vi "Test Process Broadcast Lifecycle Changes.vi"(8 "error in (no error)":errorcluster, 11 "Process Test In":refnum<class "Process Dev Test.lvclass">) -> (0 "error out":errorcluster, 3 "Process Test Out":refnum<class "Process Dev Test.lvclass">)   [LabVIEW 2020, in "Process Dev Test.lvclass"]
uses:
  Process Dev Test.lvclass
  C:/Program Files (x86)/National Instruments/LabVIEW 2020/vi.lib/Astemes/LUnit/Test Case.lvclass
  source/Framework/Process/Process.lvclass/Process.ctl
  <vilib>/Astemes/LUnit/Test Case.lvclass/Test Case.ctl
  <vilib>/Astemes/LUnit/LUnit Assertion Result.lvclass/LUnit Assertion Result.ctl
  <vilib>/Astemes/LUnit/LUnit Test Case Result.lvclass/LUnit Test Case Result.ctl
  <vilib>/Astemes/LUnit/LUnit Method Result.lvclass/LUnit Method Result.ctl
  source/Framework/Process/Public/Lifecycle/Get Lifecycle State.vi
  source/Framework/Broadcast Event Helpers/Execution timer.vi
  <vilib>/Astemes/LUnit/Palette/Fail.vi
  <vilib>/Astemes/LUnit/Palette/Pass.vi
  <vilib>/Astemes/LUnit/Set Assertion Type.vi
  source/Framework/Process/Private/SubVIs/Wait for finish.vi
  source/Framework/Process/Protected/Messaging/Enqueue Message.vi
  source/Framework/Process/Private/SubVIs/Set Lifecycle State.vi
  <vilib>/Utility/error.llb/Clear Errors.vi
  <vilib>/Astemes/LUnit/Add test result.vi
  <vilib>/Astemes/LUnit/LUnit Write Passed.vi
  <vilib>/Astemes/LUnit/LUnit Write Message.vi
  <vilib>/Astemes/LUnit/LUnit Write Description.vi
  <vilib>/Astemes/LUnit/LUnit Write Assertion Type.vi
  source/Framework/Process/Private/SubVIs/Handle Debug Data.vi
  <vilib>/Astemes/LUnit/LUnit Record Assertion Result.vi
  source/Framework/Logging/Log Debug.vi
  <vilib>/AdvancedString/1D String Array to Delimited String.vi
  <vilib>/Utility/High Resolution Relative Seconds.vi
  <vilib>/Astemes/LUnit/LUnit Aggregate Assertion Results.vi
  <vilib>/Astemes/LUnit/Assertion Result/LUnit Read Status.vi
  <vilib>/Astemes/LUnit/LUnit Read Message.vi
  <vilib>/Astemes/LUnit/LUnit Read Description.vi
  <vilib>/Astemes/LUnit/Method Result/LUnit Merge Status.vi
  <vilib>/Astemes/LUnit/LUnit Concatenate result strings.vi
  <vilib>/Utility/error.llb/Error Cluster From Error Code.vi
  source/Framework/Broadcast Event Helpers/Dequeue Broadcast Message.vi
  source/Framework/Process/Public/Read Name.vi
  <vilib>/Astemes/LUnit/LUnit Assertion Result.lvclass
  source/Framework/Process/Process.lvclass
  <vilib>/Astemes/LUnit/Test Case.lvclass
  source/Framework/Broadcast Event Helpers/Broadcast Event Helpers.lvlib
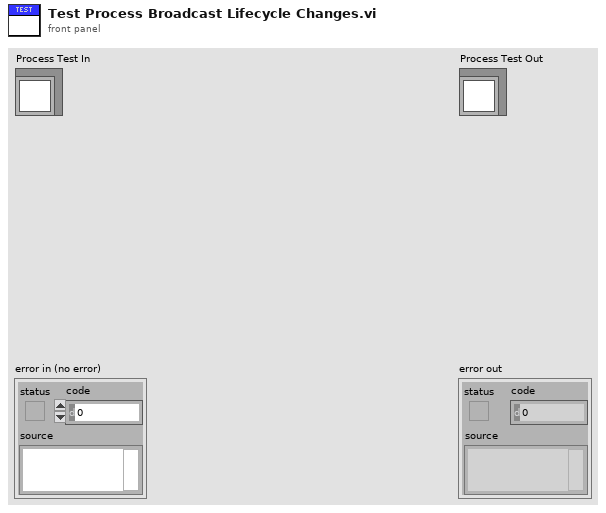
[diagram p1: front panel]
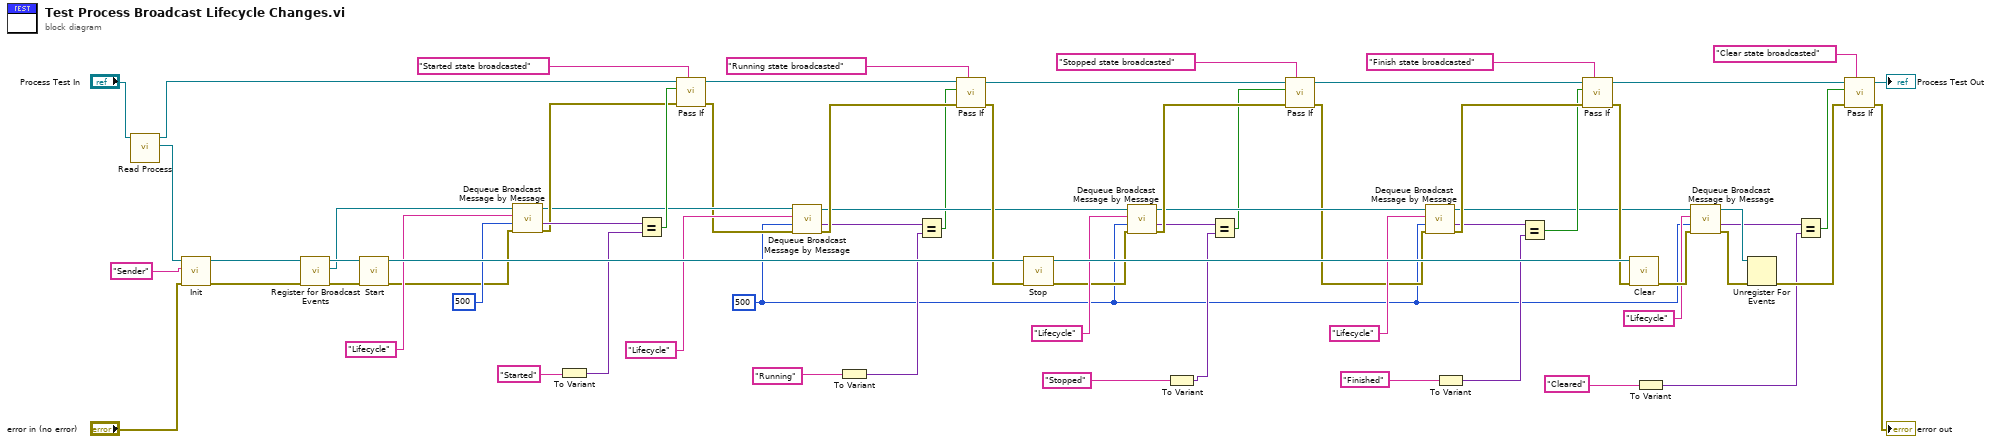
[diagram p0: block diagram]
diagram:
  w1 = 500
  n1 = call "Read Process.vi"("Process Test in"="Process Test In") -> ("Process.lvclass"=w62:refnum<class "Process.lvclass">, "Process Test out"=w21:refnum<class "Process Dev Test.lvclass">)  [unwired: 8 in, 1 out]
  n2 = call-dynamic "Init.vi"("error in (no error)"="error in (no error)", "Name"="Sender" ("Message"), "Process In"=w62) -> ("error out"=w67:errorcluster, "Process Out"=w68:refnum<class "Process.lvclass">)  [unwired: 7 in]
  n3 = call "Register for Broadcast Events.vi"("error in (no error)"=w67, "Process In"=w68) -> ("error out"=w60:errorcluster, "Event Registration Refnum Out"=w25:refnum<event-registration>, "Process Out"=w61:refnum<class "Process.lvclass">)  [unwired: 7 in]
  n4 = call "Start.vi"("error in (no error)"=w60, "Process In"=w61) -> ("error out"=w23:errorcluster, "Process Out"=w59:refnum<class "Process.lvclass">)  [unwired: 7 in, 1 out]
  n5 = call "Dequeue Broadcast Message by Message.vi"("error in (no error)"=w23, "Timeout (-1)"=500, "Message"="Lifecycle", "Event Registration Refnum"=w25) -> ("error out"=w27:errorcluster, "Message Data"=w28:variant, "Event Registration Refnum Out"=w24:refnum<event-registration>)  [unwired: 3 in, 2 out]
  n6 = To Variant(anything="Started") -> (Variant=w32:variant)
  n7 = Equal?(x=w28, y=w32) -> (x = y?=w31:bool)
  n8 = call <vilib>:"Pass If.vi"("Description"="Started state broadcasted", "error in (no error)"=w27, "Pass?"=w31, "LUnit Test Case In"=w21) -> ("error out"=w22:errorcluster, "LUnit Test Case Out"=w20:refnum<class "Process Dev Test.lvclass">)  [unwired: 6 in]
  n9 = call "Dequeue Broadcast Message by Message.vi"("error in (no error)"=w22, "Timeout (-1)"=w1, "Message"="Lifecycle", "Event Registration Refnum"=w24) -> ("error out"=w57:errorcluster, "Message Data"=w55:variant, "Event Registration Refnum Out"=w45:refnum<event-registration>)  [unwired: 3 in, 2 out]
  n10 = To Variant(anything="Running" ("Message")) -> (Variant=w38:variant)
  n11 = Equal?(x=w55, y=w38) -> (x = y?=w39:bool)
  n12 = call <vilib>:"Pass If.vi"("Description"="Running state broadcasted", "error in (no error)"=w57, "Pass?"=w39, "LUnit Test Case In"=w20) -> ("error out"=w56:errorcluster, "LUnit Test Case Out"=w41:refnum<class "Process Dev Test.lvclass">)  [unwired: 6 in]
  n13 = call "Stop.vi"("error in (no error)"=w56, "Process In"=w59) -> ("error out"=w43:errorcluster, "Process Out"=w66:refnum<class "Process.lvclass">)  [unwired: 7 in, 1 out]
  n14 = call "Dequeue Broadcast Message by Message.vi"("error in (no error)"=w43, "Timeout (-1)"=w1, "Message"="Lifecycle", "Event Registration Refnum"=w45) -> ("error out"=w49:errorcluster, "Message Data"=w47:variant, "Event Registration Refnum Out"=w44:refnum<event-registration>)  [unwired: 3 in, 2 out]
  n15 = To Variant(anything="Stopped" ("Message")) -> (Variant=w36:variant)
  n16 = Equal?(x=w47, y=w36) -> (x = y?=w37:bool)
  n17 = call <vilib>:"Pass If.vi"("Description"="Stopped state broadcasted", "error in (no error)"=w49, "Pass?"=w37, "LUnit Test Case In"=w41) -> ("error out"=w42:errorcluster, "LUnit Test Case Out"=w40:refnum<class "Process Dev Test.lvclass">)  [unwired: 6 in]
  n18 = call "Dequeue Broadcast Message by Message.vi"("error in (no error)"=w42, "Timeout (-1)"=w1, "Message"="Lifecycle", "Event Registration Refnum"=w44) -> ("error out"=w51:errorcluster, "Message Data"=w35:variant, "Event Registration Refnum Out"=w15:refnum<event-registration>)  [unwired: 3 in, 2 out]
  n19 = To Variant(anything="Finished" ("Message")) -> (Variant=w34:variant)
  n20 = Equal?(x=w35, y=w34) -> (x = y?=w33:bool)
  n21 = call <vilib>:"Pass If.vi"("Description"="Finish state broadcasted", "error in (no error)"=w51, "Pass?"=w33, "LUnit Test Case In"=w40) -> ("error out"=w50:errorcluster, "LUnit Test Case Out"=w11:refnum<class "Process Dev Test.lvclass">)  [unwired: 6 in]
  n22 = call-dynamic "Clear.vi"("error in (no error)"=w50, "Process In"=w66) -> ("error out"=w14:errorcluster)  [unwired: 9 in]
  n23 = To Variant(anything="Cleared" ("Message")) -> (Variant=w4:variant)
  n24 = call "Dequeue Broadcast Message by Message.vi"("error in (no error)"=w14, "Timeout (-1)"=w1, "Message"="Lifecycle", "Event Registration Refnum"=w15) -> ("error out"=w13:errorcluster, "Message Data"=w5:variant, "Event Registration Refnum Out"=w12:refnum<event-registration>)  [unwired: 3 in, 2 out]
  n25 = Unregister For Events(event registration refnum=w12, error in=w13) -> (error out=w9:errorcluster)
  n26 = Equal?(x=w5, y=w4) -> (x = y?=w3:bool)
  n27 = call <vilib>:"Pass If.vi"("Description"="Clear state broadcasted", "error in (no error)"=w9, "Pass?"=w3, "LUnit Test Case In"=w11) -> ("error out"=→"error out":errorcluster, "LUnit Test Case Out"=→"Process Test Out":refnum<class "Process Dev Test.lvclass">)  [unwired: 6 in]
